vi "Sync Pulse.vi"(9 "Pulse duration (ticks)":u32=4, 11 "Sync":bool) -> (3 "Sync Enable?":bool)   [LabVIEW 2015, in "Engine Simulation Toolkit.lvlib" / "APU.lvlib"]
doc: "Sets <b>Sync Enable?</b> to true for the specified duration once <b>Sync</b> is set to true. This assumes <b>Sync</b> is set to latch so it is only true for one cycle."
uses:
  APU.lvlib
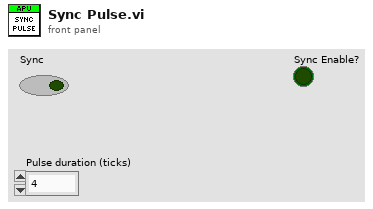
[diagram p1: front panel]
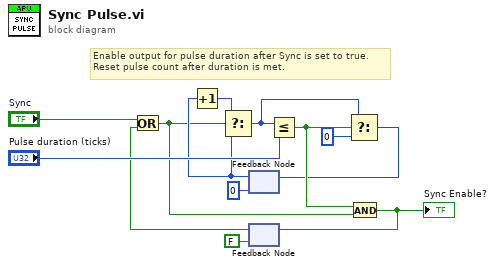
[diagram p0: block diagram]
diagram:
  # "Enable output for pulse duration after Sync is set to true.\nReset pulse count after duration is met."
  n1 = feedback #1(u32 0) -> (w11:u32)
  n2 = Increment(x=w11) -> (x+1=w12:u32)
  n3 = feedback #2(FALSE) -> (w9:bool)
  n4 = Or(x="Sync", y=w9) -> (x .or. y?=w5:bool)
  n5 = Select(t=w12, s=w5, f=w11) -> (s? t:f=w7:u32)
  n6 = Less Or Equal?(x=w7, y="Pulse duration (ticks)") -> (x <= y?=w4:bool)
  n7 = Select(t=w7, s=w4, f=u32 0) -> (s? t:f=w1:u32)
  n8 = feedback-in #1(w1) -> ()
  n9 = And(x=w4, y=w5) -> (x .and. y?=w2:bool)
  "Sync Enable?" <- w2
  n10 = feedback-in #2(w2) -> ()
